vi "EVM_Sweep_Only_R_S_CMP200.vi"() -> ()   [LabVIEW 2023, in "EVM.lvlib"]
uses:
  lib/CTL/LitePoint_EVM_SG.ctl
  lib/CTL/LitePoint_EVM_SA.ctl
  EVM.lvlib
  lib/LitePoints/LitePoints.lvlib
  lib/FTDI/JIO/CLC_JIO_FTDI.lvlib
  lib/R_S/R_S.lvlib
panel:
  out "ReceivedPower":dbl format="%#.3g"
  out "Best EVM ALL":dbl
  out "PST(sec)":dbl
  out "Best EVM":dbl
  out "error out":errorcluster
  in  "Power res":i32=2
  in  "Stop Power":i32
  in  "Start Power":i32=-40
  in  "BFIC_ele_stop":i32=12
  in  "BFIC_ele_res":i32=4
  in  "BFIC_ele_start":i32
  in  "BFIC_com_stop":i32=12
  in  "BFIC_com_res":i32=4
  in  "BFIC_com_start":i32
  in  "UD_att_stop":i32=120
  in  "UD_att_res":i32=8
  in  "UD_att_start":i32
  out "UD_att":i32=255
  out "BFIC_com_step":i32=15
  out "BFIC_ele_step":i32=15
  out "SG Power":i32=-10
  in  "TRXmode":u16(ring)=1 items=["Tx"=1, "Rx"=2]
  in  "Polarity":u16(ring) items=["H", "V"]
  out "floder Exist?":bool=TRUE
  in  "Waiting \nTime(ms)":u32=1
  in  "FileNote":string="test16_wayne_MCS11"
  in  "SG":refnum<visa-resource-name>="TCPIP::192.168.88.12::hislip0::INSTR"
  in  "SA":refnum<visa-resource-name>="TCPIP0::LAB_XBeam-NB::inst0::INSTR"
  out "Spectrum Data":cluster{"X":dbl, "Y":dbl}[](graph)
  # "TMYTEK_CLC_JIO_R&S_EVM"
  # "12"
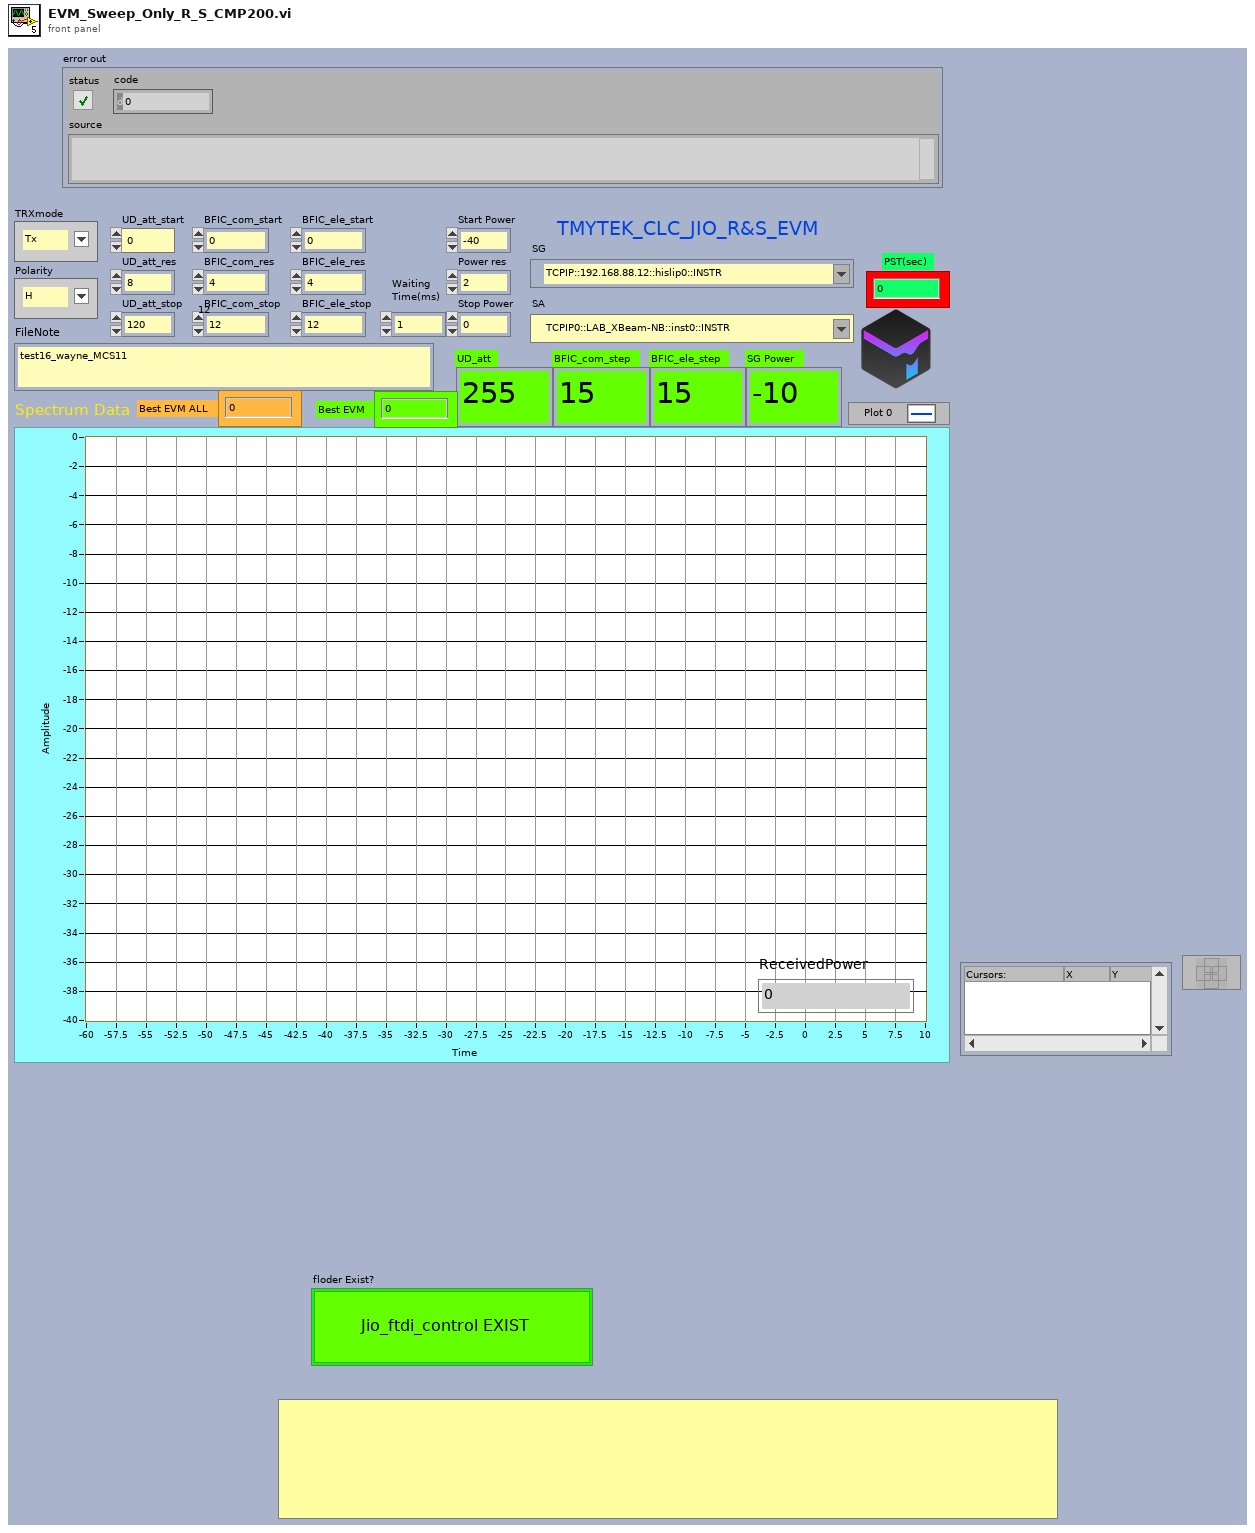
[diagram p1: front panel]
types:
  T1 = typedef "LitePoint_EVM_SG.ctl" = enum16{"Init", "Close", "set_SG", "AdjustLevel", "byPass", "RF_ON", "RF_OFF"}
  T2 = typedef "LitePoint_EVM_SA.ctl" = enum16{"Init", "Close", "set_SA", "get_EVM", "byPass", "getPower"}
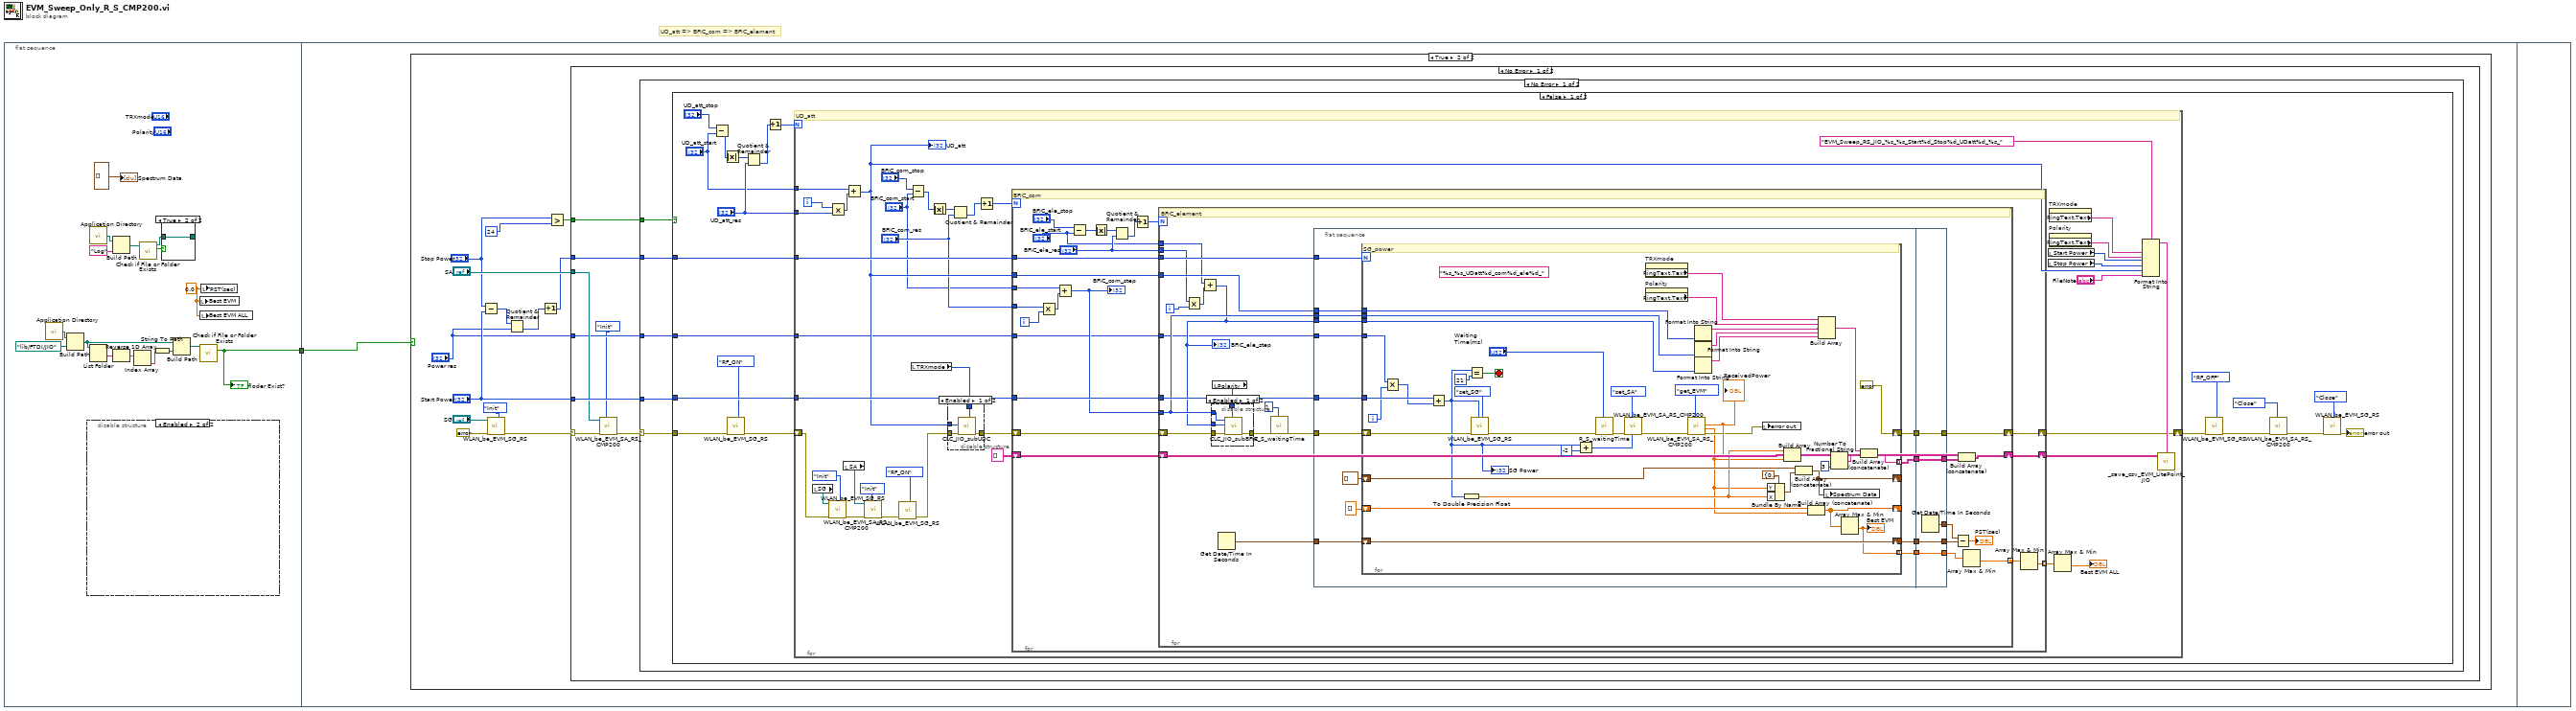
[diagram p0: block diagram]
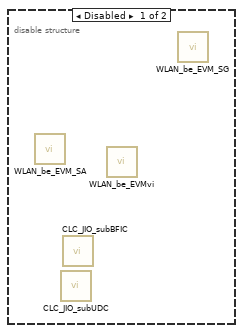
[diagram p2: hidden frame]
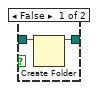
[diagram p3: hidden frame]
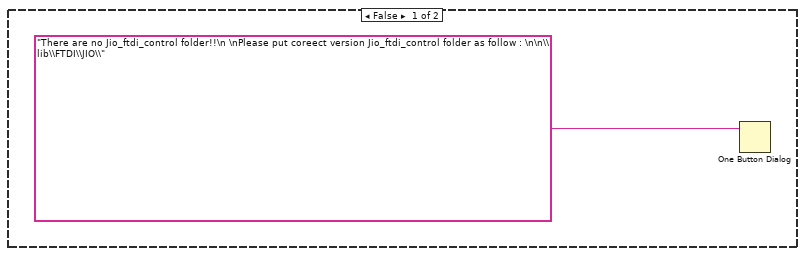
[diagram p4: hidden frame]
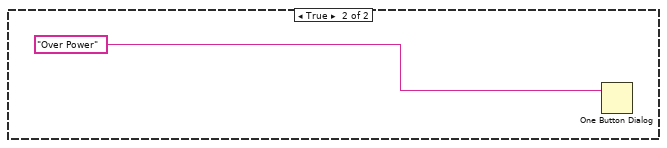
[diagram p7: hidden frame]
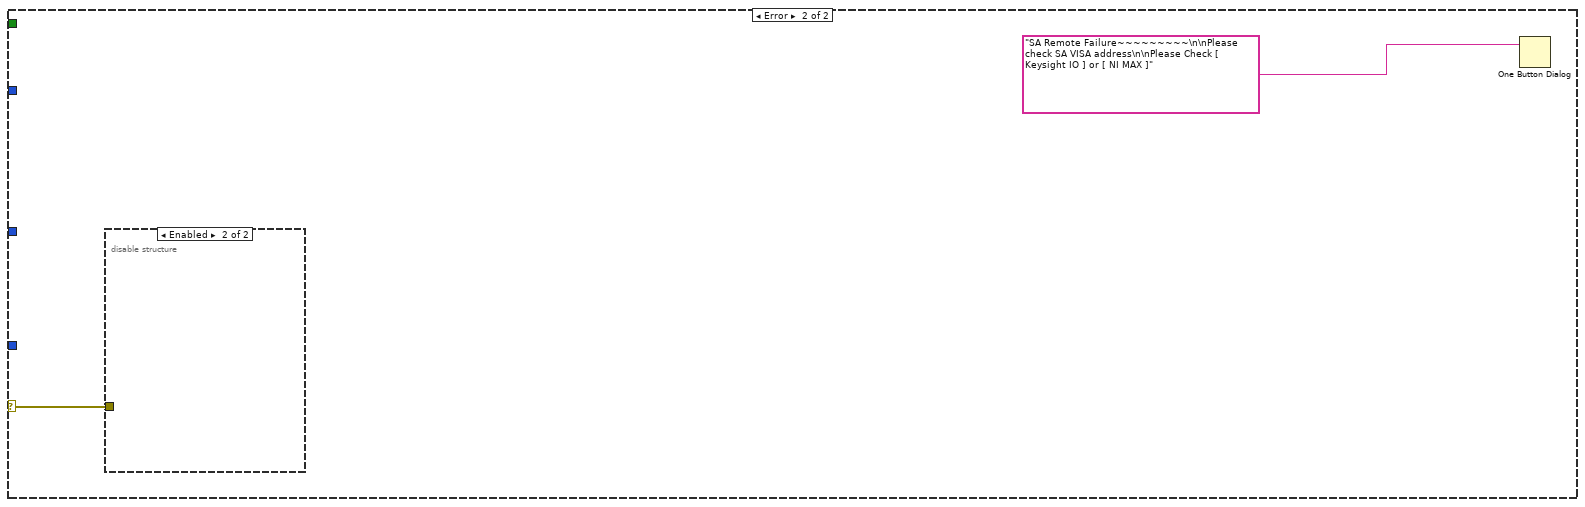
[diagram p8: hidden frame]
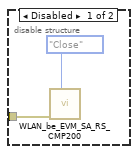
[diagram p9: hidden frame]
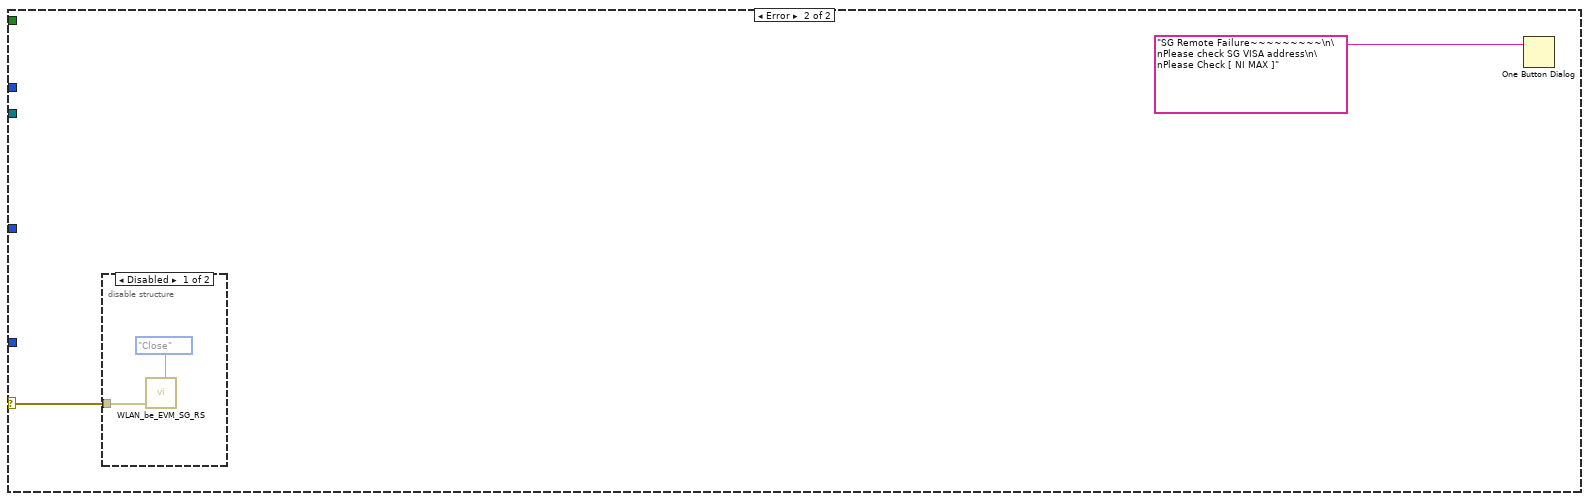
[diagram p10: hidden frame]
diagram:
  # "UD_att => BFIC_com => BFIC_element"
  n1 = flat-sequence {
    tunnel: [w3] -> w1
    tunnel: w1 -> [w21]
    frame #0 {
      w2 = 0.0 ("PST(sec)")
      n2 = call <vilib>:"Application Directory.vi"() -> ("Application Directory"=w9:path)
      n3 = Build Path(base path=w9, name or relative path=path "lib/FTDI/JIO") -> (appended path=w10:path)
      n4 = disable-structure shown="Enabled" {
        frame Disabled {
          n5 = call "WLAN_be_EVM_SA.vi"() -> ()  [unwired: 8 in, 4 out]
          n6 = call "CLC_JIO_subUDC.vi"() -> ()  [unwired: 10 in, 2 out]
          n7 = call "CLC_JIO_subBFIC.vi"() -> ()  [unwired: 10 in, 2 out]
          n8 = call "WLAN_be_EVMvi.vi"() -> ()  [unwired: 8 in, 4 out]
          n9 = call "WLAN_be_EVM_SG.vi"() -> ()  [unwired: 10 in, 2 out]
        }
        frame Enabled {
        }
      }
      n10 = call <vilib>:"Application Directory.vi"() -> ("Application Directory"=w16:path)
      n11 = List Folder(path=w10) -> (folder names=w5:string[])  [unwired: 3 in, 3 out]
      n12 = Reverse 1D Array(array=w5) -> (reversed array=w6:string[])
      n13 = Build Path(base path=w16, name or relative path="Log") -> (appended path=w13:path)
      n14 = Index Array(array=w6) -> (element=w7:string)  [unwired: 1 in]
      n15 = call <vilib>:"Check if File or Folder Exists.vi"("path"=w13) -> ("file or folder exists?"=w15:bool, "dup path"=w14:path)  [unwired: 8 in, 1 out]
      n16 = String To Path(string=w7) -> (path=w8:path)
      n17 = case shown="True" w15 {
        tunnel: w14 -> [w19 w20]
        tunnel: [w18 w20] -> _
        frame False {
          n18 = Create Folder(path (use dialog)=w19) -> (created path=w18:path)  [unwired: 2 in, 2 out]
        }
        frame True {
        }
      }
      n19 = Build Path(base path=w10, name or relative path=w8) -> (appended path=w11:path)
      n20 = local write "Best EVM"(w2) -> ()
      n21 = local write "Best EVM ALL"(w2) -> ()
      n22 = call <vilib>:"Check if File or Folder Exists.vi"("path"=w11) -> ("file or folder exists?"=w3:bool)  [unwired: 8 in, 2 out]
      "floder Exist?" <- w3
      n23 = local write "PST(sec)"(w2) -> ()
      "Spectrum Data" <- cluster{"X":dbl, "Y":dbl}[] [] ("XY Graph")
    }
    frame #1 {
      n24 = case shown="True" w21 {
        frame False {
          n25 = One Button Dialog(message="There are no Jio_ftdi_control folder!!\n \nPlease put coreect version Jio_ftdi_control folder as follow : \n\n\\lib\\FTDI\\JIO\\") -> ()  [unwired: 1 in, 1 out]
        }
        frame True {
          n26 = Subtract(x="Stop Power", y="Start Power") -> (x-y=w26:i32)
          n27 = call "WLAN_be_EVM_SG_RS.vi"("Function_SG"=LitePoint_EVM_SG."Init", "error in"=errorcluster {"status"=FALSE, "code"=0, "source"=""} ("error in (no error)"), "VISA IN"="SG") -> ("error out"=w28:errorcluster)  [unwired: 7 in, 1 out]
          n28 = Quotient & Remainder(x=w26, y="Power res") -> (floor(x/y)=w25:i32)  [unwired: 1 out]
          n29 = Increment(x=w25) -> (x+1=w32:i32)
          n30 = Greater?(x="Stop Power", y=24) -> (0:w34:bool)
          n31 = case shown="No Error" w28 {
            selector: w28 -> [w40 w236]
            tunnel: "SA" -> [w38 _]
            tunnel: w34 -> [w43 _]
            tunnel: "Start Power" -> [w42 _]
            tunnel: w32 -> [w41 _]
            tunnel: "Power res" -> [w37 _]
            frame No Error {
              n32 = call "WLAN_be_EVM_SA_RS_CMP200.vi"("Function"=LitePoint_EVM_SA."Init", "error in"=w40, "VISA IN"=w38) -> ("error out"=w39:errorcluster)  [unwired: 5 in, 3 out]
              n33 = case shown="No Error" w39 {
                selector: w39 -> [w45 w232]
                tunnel: w43 -> [w48 _]
                tunnel: w42 -> [w47 _]
                tunnel: w41 -> [w46 _]
                tunnel: w37 -> [w44 _]
                frame No Error {
                  n34 = case shown="False" w48 {
                    tunnel: w47 -> [w67 _]
                    tunnel: w45 -> [w66 _]
                    tunnel: w46 -> [w68 _]
                    tunnel: w44 -> [w54 _]
                    frame False {
                      n35 = Subtract(x="UD_att_stop", y="UD_att_start") -> (x-y=w61:i32)
                      n36 = Absolute Value(x=w61) -> (abs(x)=w58:i32)
                      n37 = call "WLAN_be_EVM_SG_RS.vi"("Function_SG"=LitePoint_EVM_SG."RF_ON", "error in"=w66) -> ("error out"=w64:errorcluster)  [unwired: 8 in, 1 out]
                      n38 = Quotient & Remainder(x=w58, y="UD_att_res") -> (floor(x/y)=w59:i32)  [unwired: 1 out]
                      n39 = Increment(x=w59) -> (x+1=w55:i32)
                      n40 = for {
                        N: w55 -> [_]
                        tunnel: w68 -> [w106]
                        tunnel: w67 -> [w105]
                        shift-right: [w93] -> w63
                        shift-left: w64 -> [w78]
                        tunnel: "UD_att_res" -> [w90]
                        tunnel: "UD_att_start" -> [w89]
                        tunnel: w54 -> [w80]
                        i -> [w92]
                        # "UD_att"
                        n41 = local read "SG"() -> (w75:refnum<visa-resource-name>)
                        n42 = call "WLAN_be_EVM_SG_RS.vi"("Function_SG"=LitePoint_EVM_SG."Init", "error in"=w78, "VISA IN"=w75) -> ("error out"=w76:errorcluster)  [unwired: 7 in, 1 out]
                        n43 = Multiply(x=w92, y=w90) -> (x*y=w91:i32)
                        n44 = local read "SA"() -> (w74:refnum<visa-resource-name>)
                        n45 = Add(x=w89, y=w91) -> (x+y=w88:i32)
                        "UD_att" <- w88
                        n46 = call "WLAN_be_EVM_SA_RS_CMP200.vi"("Function"=LitePoint_EVM_SA."Init", "error in"=w76, "VISA IN"=w74) -> ("error out"=w72:errorcluster)  [unwired: 5 in, 3 out]
                        n47 = call "WLAN_be_EVM_SG_RS.vi"("Function_SG"=LitePoint_EVM_SG."RF_ON", "error in"=w72) -> ("error out"=w71:errorcluster)  [unwired: 8 in, 1 out]
                        n48 = Subtract(x="BFIC_com_stop", y="BFIC_com_start") -> (x-y=w87:i32)
                        n49 = local read "TRXmode"() -> (w102:u16)
                        n50 = Absolute Value(x=w87) -> (abs(x)=w86:i32)
                        n51 = disable-structure shown="Enabled" {
                          disable-tunnel: [w110 w111] -> w104
                          disable-tunnel: w71 -> [w109 w111]
                          disable-tunnel: w102 -> [w108 _]
                          disable-tunnel: w88 -> [w107 _]
                          frame Enabled {
                            n52 = call "CLC_JIO_subUDC.vi"("Mode"=w108, "error in"=w109, "ud att"=w107) -> ("error out"=w110:errorcluster)  [unwired: 7 in, 1 out]
                          }
                          frame Disabled {
                          }
                        }
                        n53 = Quotient & Remainder(x=w86, y="BFIC_com_res") -> (floor(x/y)=w82:i32)  [unwired: 1 out]
                        n54 = Increment(x=w82) -> (x+1=w81:i32)
                        n55 = for {
                          N: w81 -> [_]
                          tunnel: w106 -> [w133]
                          tunnel: w105 -> [w132]
                          shift-right: [w129] -> w103
                          shift-left: string[][] [] -> [w130]
                          tunnel: w88 -> [w128]
                          shift-right: [w127] -> w93
                          shift-left: w104 -> [w131]
                          tunnel: "BFIC_com_res" -> [w123]
                          tunnel: "BFIC_com_start" -> [w122]
                          tunnel: w80 -> [w114]
                          tunnel: [w112] -> w70 mode=indexing
                          i -> [w125]
                          # "BFIC_com"
                          n56 = Multiply(x=w123, y=w125) -> (x*y=w126:i32)
                          n57 = Add(x=w122, y=w126) -> (x+y=w124:i32)
                          "BFIC_com_step" <- w124
                          n58 = Subtract(x="BFIC_ele_stop", y="BFIC_ele_start") -> (x-y=w120:i32)
                          n59 = Absolute Value(x=w120) -> (abs(x)=w121:i32)
                          n60 = Quotient & Remainder(x=w121, y="BFIC_ele_res") -> (floor(x/y)=w118:i32)  [unwired: 1 out]
                          n61 = Increment(x=w118) -> (x+1=w115:i32)
                          n62 = for {
                            N: w115 -> [_]
                            tunnel: w133 -> [w162]
                            tunnel: w132 -> [w161]
                            shift-right: [w159] -> w129
                            shift-left: w130 -> [w158]
                            tunnel: w124 -> [w153]
                            tunnel: w128 -> [w154]
                            shift-right: [w137] -> w127
                            shift-left: w131 -> [w157]
                            tunnel: "BFIC_ele_res" -> [w148]
                            tunnel: "BFIC_ele_start" -> [w147]
                            tunnel: w114 -> [w146]
                            tunnel: [w134] -> w113 mode=indexing
                            i -> [w149]
                            # "BFIC_element"
                            n63 = Multiply(x=w148, y=w149) -> (x*y=w151:i32)
                            n64 = Add(x=w147, y=w151) -> (x+y=w150:i32)
                            "BFIC_ele_step" <- w150
                            n65 = local read "Polarity"() -> (w152:u16)
                            n66 = disable-structure shown="Enabled" {
                              disable-tunnel: w157 -> [w229 w230]
                              disable-tunnel: [w228 w230] -> w156
                              disable-tunnel: w150 -> [w227 _]
                              disable-tunnel: w153 -> [w226 _]
                              disable-tunnel: w152 -> [w225 _]
                              frame Enabled {
                                n67 = call "CLC_JIO_subBFIC.vi"("pol"=w225, "error in"=w229, "ele"=w227, "com"=w226) -> ("error out"=w228:errorcluster)  [unwired: 6 in, 1 out]
                              }
                              frame Disabled {
                              }
                            }
                            n68 = Get Date/Time In Seconds() -> (seconds since 1Jan1904=w144:timestamp)
                            n69 = call "R_S_waitingTime.vi"("Waiting Time(ms)"=u32 1, "error in"=w156) -> ("error out"=w145:errorcluster)  [unwired: 9 in]
                            n70 = flat-sequence {
                              tunnel: w162 -> [w176]
                              tunnel: w161 -> [w174]
                              tunnel: w154 -> [w172]
                              tunnel: w153 -> [w171]
                              tunnel: w150 -> [w169]
                              tunnel: w146 -> [w168]
                              tunnel: w145 -> [w167]
                              tunnel: w144 -> [w165]
                              tunnel: [w173] -> w142
                              tunnel: [w170] -> w141
                              tunnel: [w164] -> w140
                              tunnel: [w163] -> w136
                              tunnel: [w222] -> w143
                              tunnel: [w223] -> w137
                              tunnel: [w224] -> w160
                              tunnel: w142 -> [w224]
                              tunnel: w141 -> [w223]
                              tunnel: w140 -> [w222]
                              tunnel: [w221] -> w139
                              tunnel: [w220] -> w135
                              tunnel: w136 -> [w220]
                              frame #0 {
                                n71 = for {
                                N: w176 -> [_]
                                tunnel: w174 -> [w219]
                                shift-right: [errorcluster {"status"=FALSE, "code"=0, "source"=""} ("error out")] -> w170
                                shift-left: w167 -> [w211]
                                shift-right: [w213] -> _
                                shift-left: cluster{"X":dbl, "Y":dbl}[] [] ("XY Graph") -> [w215]
                                tunnel: [w203] -> w173 mode=indexing
                                tunnel: w172 -> [w200]
                                tunnel: w169 -> [w198]
                                tunnel: w171 -> [w199]
                                tunnel: w168 -> [w192]
                                shift-right: [w180] -> _
                                shift-left: dbl[] [] -> [w182]
                                shift-right: [w179] -> w164
                                shift-left: w165 -> [w179]
                                tunnel: [w177] -> w163 mode=indexing
                                i -> [w193]
                                stop <- w217 stop-if-true
                                (unwired) "%s_%s_UDatt%d_com%d_ele%d_" ("format string")
                                # "SG_power"
                                n72 = Multiply(x=w192, y=w193) -> (x*y=w191:i32)
                                n73 = Add(x=w219, y=w191) -> (x+y=w185:i32)
                                "SG Power" <- w185
                                n74 = To Double Precision Float(number=w185) -> (double precision float=w212:dbl)
                                n75 = Equal?(x=w185, y=21) -> (x = y?=w217:bool)
                                n76 = call "WLAN_be_EVM_SG_RS.vi"("Function_SG"=LitePoint_EVM_SG."set_SG", "setPower"=w185, "error in"=w211) -> ("error out"=w189:errorcluster)  [unwired: 7 in, 1 out]
                                n77 = Add(x=w185, y=-2) -> (x+y=w184:i32)
                                n78 = call "R_S_waitingTime.vi"("Waiting Time(ms)"="Waiting \nTime(ms)", "error in"=w189) -> ("error out"=w207:errorcluster)  [unwired: 9 in]
                                n79 = call "WLAN_be_EVM_SA_RS_CMP200.vi"("SG Power"=w184, "Function"=LitePoint_EVM_SA."set_SA", "error in"=w207) -> ("error out"=w187:errorcluster)  [unwired: 5 in, 3 out]
                                n80 = property on="TRXmode" class="Ring (strict)"() -> ("RingText.Text"=w202:string)  [unwired: 2 in, 2 out]
                                n81 = property on="Polarity" class="Ring (strict)"() -> ("RingText.Text"=w201:string)  [unwired: 2 in, 2 out]
                                n82 = call "WLAN_be_EVM_SA_RS_CMP200.vi"("Function"=LitePoint_EVM_SA."get_EVM", "error in"=w187) -> ("error out"=w186:errorcluster, "EVM"=w181:dbl, "Power"=w190:dbl)  [unwired: 6 in, 1 out]
                                "ReceivedPower" <- w190
                                n83 = Format Into String(w200) -> (resulting string=w197:string)  [unwired: 3 in, 1 out]
                                n84 = Format Into String(w199) -> (resulting string=w196:string)  [unwired: 3 in, 1 out]
                                n85 = Format Into String(w198) -> (resulting string=w195:string)  [unwired: 3 in, 1 out]
                                n86 = local write "error out"(w186) -> ()
                                n87 = Bundle By Name(cluster=cluster{"X":dbl, "Y":dbl} {"X"=0.0, "Y"=0.0} ("element"), "Y"=w181, "X"=w212) -> (w214:cluster{"X":dbl, "Y":dbl})
                                n88 = Build Array(w212, w190, w181) -> (w205:dbl[])
                                n89 = Build Array (concatenate)(w215, w214) -> (w213:cluster{"X":dbl, "Y":dbl}[])
                                n90 = Build Array (concatenate)(w182, w181) -> (w180:dbl[])
                                n91 = Build Array(w202, w201, w197, w196, w195) -> (w194:string[])
                                n92 = local write "Spectrum Data"(w213) -> ()
                                n93 = Number To Fractional String(number=w205, precision (6)=i16 3) -> (F-format string=w204:string[])  [unwired: 2 in]
                                n94 = Array Max & Min(array=w180) -> (min value=w177:dbl)  [unwired: 3 out]
                                "Best EVM" <- w177
                                n95 = Build Array (concatenate)(w194, w204) -> (w203:string[])
                                }
                              }
                              frame #1 {
                                n96 = Get Date/Time In Seconds() -> (seconds since 1Jan1904=w221:timestamp)
                              }
                            }
                            n97 = Subtract(x=w139, y=w143) -> (x-y=→"PST(sec)":dbl)
                            n98 = Build Array (concatenate)(w158, w160) -> (w159:string[][])
                            n99 = Array Max & Min(array=w135) -> (min value=w134:dbl)  [unwired: 3 out]
                          }
                          n100 = Array Max & Min(array=w113) -> (min value=w112:dbl)  [unwired: 3 out]
                        }
                        n101 = local read "Start Power"() -> (w97:i32)
                        n102 = local read "Stop Power"() -> (w99:i32)
                        n103 = property on="TRXmode" class="Ring (strict)"() -> ("RingText.Text"=w95:string)  [unwired: 2 in, 2 out]
                        n104 = property on="Polarity" class="Ring (strict)"() -> ("RingText.Text"=w96:string)  [unwired: 2 in, 2 out]
                        n105 = Array Max & Min(array=w70) -> (min value=→"Best EVM ALL":dbl)  [unwired: 3 out]
                        n106 = Format Into String(format string="EVM_Sweep_RS_JIO_%s_%s_Start%d_Stop%d_UDatt%d_%s_" ("delimiter (\\t)"), w95, w96, w97, w99, w88, "FileNote") -> (resulting string=w100:string)  [unwired: 2 in, 1 out]
                        n107 = call "_save_csv_EVM_LitePoint_JIO.vi"("delimiter (\\t)"=w100, "array in"=w103) -> ()  [unwired: 9 in, 1 out]
                      }
                      n108 = call "WLAN_be_EVM_SG_RS.vi"("Function_SG"=LitePoint_EVM_SG."RF_OFF", "error in"=w63) -> ("error out"=w51:errorcluster)  [unwired: 8 in, 1 out]
                      n109 = call "WLAN_be_EVM_SA_RS_CMP200.vi"("Function"=LitePoint_EVM_SA."Close", "error in"=w51) -> ("error out"=w50:errorcluster)  [unwired: 6 in, 3 out]
                      n110 = call "WLAN_be_EVM_SG_RS.vi"("Function_SG"=LitePoint_EVM_SG."Close", "error in"=w50) -> ("error out"=→"error out":errorcluster)  [unwired: 8 in, 1 out]
                    }
                    frame True {
                      n111 = One Button Dialog(message="Over Power") -> ()  [unwired: 1 in, 1 out]
                    }
                  }
                }
                frame Error {
                  n112 = disable-structure shown="Enabled" {
                    disable-tunnel: w232 -> [w235 _]
                    frame Disabled {
                      n113 = call "WLAN_be_EVM_SA_RS_CMP200.vi"("Function"=LitePoint_EVM_SA."Close", "error in"=w235) -> ()  [unwired: 6 in, 4 out]
                    }
                    frame Enabled {
                    }
                  }
                  n114 = One Button Dialog(message="SA Remote Failure~~~~~~~~~\n\nPlease check SA VISA address\n\nPlease Check [ Keysight IO ] or [ NI MAX ]") -> ()  [unwired: 1 in, 1 out]
                }
              }
            }
            frame Error {
              n115 = disable-structure shown="Disabled" {
                disable-tunnel: w236 -> [w239 _]
                frame Disabled {
                  n116 = call "WLAN_be_EVM_SG_RS.vi"("Function_SG"=LitePoint_EVM_SG."Close", "error in"=w239) -> ()  [unwired: 8 in, 2 out]
                }
                frame Enabled {
                }
              }
              n117 = One Button Dialog(message="SG Remote Failure~~~~~~~~~\n\nPlease check SG VISA address\n\nPlease Check [ NI MAX ]") -> ()  [unwired: 1 in, 1 out]
            }
          }
        }
      }
    }
    frame #2 {
    }
  }
